vi "manage_errors (SubVI).vi"(8 "Enum":T1, 9 "Temperature Array":dbl[](array[numeric]), 10 "Data in":T2) -> (1 "Boolean out":bool, 2 "Out value":dbl)   [LabVIEW 2015]
uses:
  data_typedef.ctl
  DBEnum.ctl
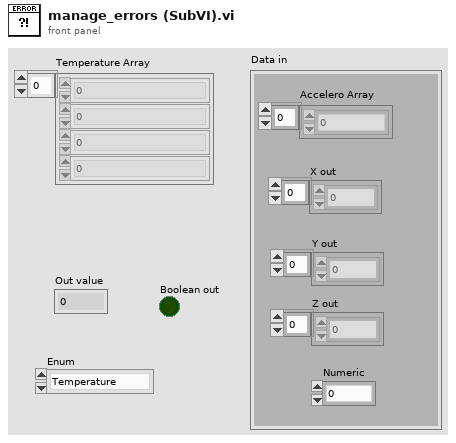
[diagram p1: front panel]
types:
  T1 = typedef "DBEnum.ctl" = enum16{"Temperature", "HeartRate", "XAccelero", "YAccelero", "ZAccelero"}
  T2 = typedef "data_typedef.ctl" = cluster{"Accelero Array":dbl[], "Z out":dbl[], "Y out":dbl[], "X out":dbl[], "Numeric":i32}
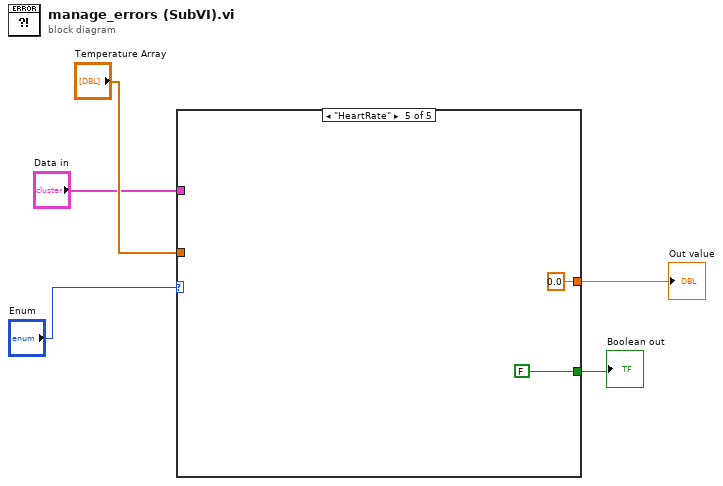
[diagram p0: block diagram]
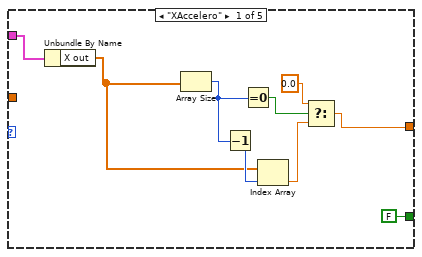
[diagram p2: hidden frame]
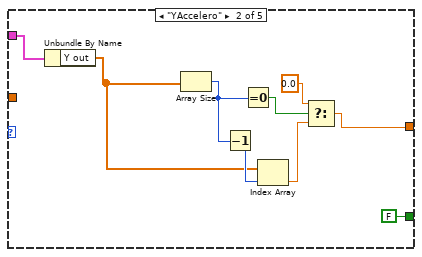
[diagram p3: hidden frame]
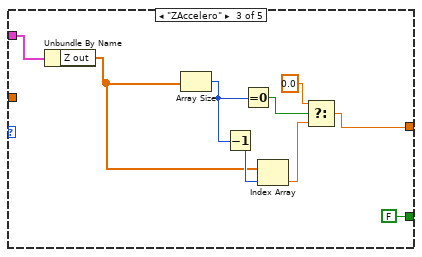
[diagram p4: hidden frame]
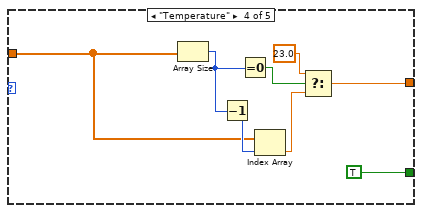
[diagram p5: hidden frame]
diagram:
  n1 = case shown="\"HeartRate\"" "Enum" {
    tunnel: [w7 w16 w25 w40 0.0 ("Numeric")] -> w5
    tunnel: [FALSE ("Boolean") FALSE ("Boolean") FALSE ("Boolean") TRUE ("Boolean") FALSE ("Boolean")] -> w4
    tunnel: "Temperature Array" -> [_ _ _ w34 _]
    tunnel: "Data in" -> [w9 w18 w27 _ _]
    frame "XAccelero" {
      n2 = Unbundle By Name(w9) -> ("X out"=w8:dbl[])
      n3 = Array Size(array=w8) -> (size(s)=w11:i32)
      n4 = Decrement(x=w11) -> (x-1=w12:i32)
      n5 = Equal To 0?(x=w11) -> (x = 0?=w14:bool)
      n6 = Index Array(array=w8, index=w12) -> (element=w10:dbl)
      n7 = Select(t=0.0, s=w14, f=w10) -> (s? t:f=w7:dbl)
    }
    frame "YAccelero" {
      n8 = Unbundle By Name(w18) -> ("Y out"=w17:dbl[])
      n9 = Array Size(array=w17) -> (size(s)=w20:i32)
      n10 = Decrement(x=w20) -> (x-1=w21:i32)
      n11 = Equal To 0?(x=w20) -> (x = 0?=w23:bool)
      n12 = Index Array(array=w17, index=w21) -> (element=w19:dbl)
      n13 = Select(t=0.0, s=w23, f=w19) -> (s? t:f=w16:dbl)
    }
    frame "ZAccelero" {
      n14 = Unbundle By Name(w27) -> ("Z out"=w26:dbl[])
      n15 = Array Size(array=w26) -> (size(s)=w29:i32)
      n16 = Decrement(x=w29) -> (x-1=w30:i32)
      n17 = Equal To 0?(x=w29) -> (x = 0?=w32:bool)
      n18 = Index Array(array=w26, index=w30) -> (element=w28:dbl)
      n19 = Select(t=0.0, s=w32, f=w28) -> (s? t:f=w25:dbl)
    }
    frame "Temperature" {
      n20 = Array Size(array=w34) -> (size(s)=w35:i32)
      n21 = Decrement(x=w35) -> (x-1=w36:i32)
      n22 = Equal To 0?(x=w35) -> (x = 0?=w38:bool)
      n23 = Index Array(array=w34, index=w36) -> (element=w33:dbl)
      n24 = Select(t=23.0, s=w38, f=w33) -> (s? t:f=w40:dbl)
    }
    frame "HeartRate" {
    }
  }
  "Out value" <- w5
  "Boolean out" <- w4
